vi "map wall setting.vi"(8 "error in (no error)":errorcluster, 11 "wall settings":cluster{"Array":cluster{"X":dbl, "Y":dbl}[]}[](array[cluster])) -> (0 "error out":errorcluster, 3 "<JSON>":string)   [LabVIEW 2019]
uses:
  <vilib>/JDP Science/JSONtext/support/Format JSON Object.vi
  <vilib>/JDP Science/JSONtext/support/Format JSON Array Text.vi
  <vilib>/JDP Science/JSONtext/JSONtext.lvlib
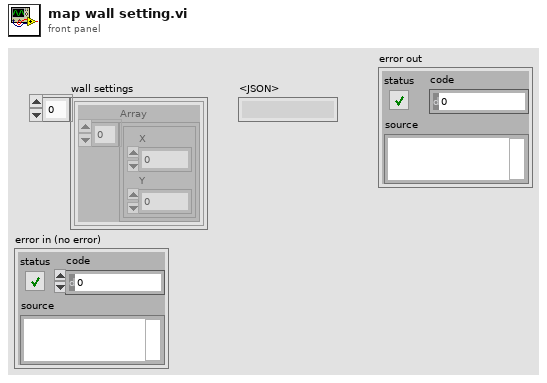
[diagram p1: front panel]
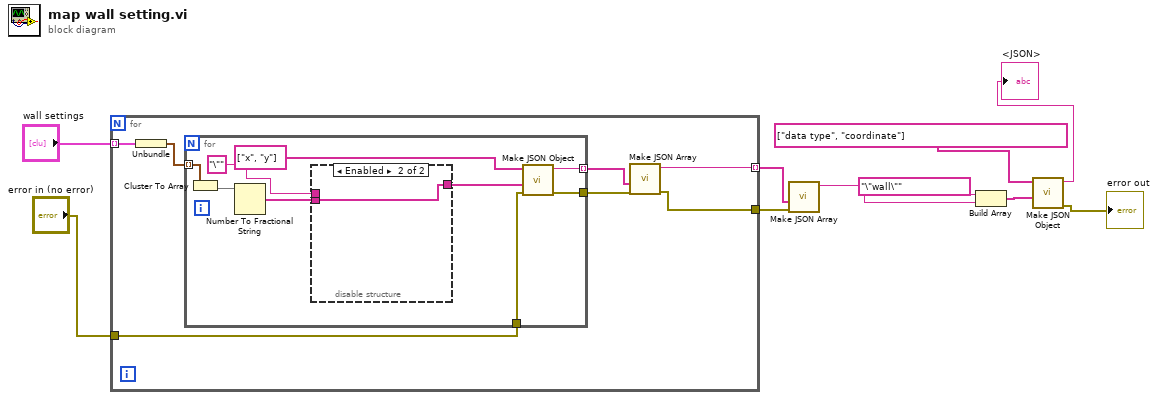
[diagram p0: block diagram]
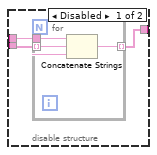
[diagram p2: hidden frame]
diagram:
  n1 = for {
    tunnel: "wall settings" -> [w17] mode=indexing
    tunnel: [w14] -> w10 mode=indexing
    tunnel: "error in (no error)" -> [w13]
    tunnel: [w11] -> w7
    n2 = Unbundle(w17) -> ("Array"=w16:cluster{"X":dbl, "Y":dbl}[])
    n3 = for {
      tunnel: w16 -> [w26] mode=indexing
      tunnel: [w23] -> w15 mode=indexing
      tunnel: w13 -> [w22]
      tunnel: [w21] -> w12
      n4 = Cluster To Array(cluster=w26) -> (array=w25:dbl[])
      n5 = Number To Fractional String(number=w25) -> (F-format string=w20:string[])  [unwired: 3 in]
      n6 = disable-structure shown="Enabled" {
        disable-tunnel: w20 -> [w29 w33]
        disable-tunnel: "\"" -> [w28 _]
        disable-tunnel: [w27 w33] -> w18
        frame Disabled {
          n7 = for {
            tunnel: w29 -> [w32] mode=indexing
            tunnel: w28 -> [w31]
            tunnel: [w30] -> w27 mode=indexing
            n8 = Concatenate Strings(w31, w32, w31) -> (w30:string)
          }
        }
        frame Enabled {
        }
      }
      n9 = call <vilib>:"Make JSON Object.vi"("error in (no error)"=w22, "JSON Items"=w18, "Item Names"=string[] ["x", "y"]) -> ("error out"=w21:errorcluster, "<JSON>"=w23:string)  [unwired: 7 in]
    }
    n10 = call <vilib>:"Make JSON Array.vi"("error in (no error)"=w12, "JSON Elements"=w15) -> ("error out"=w11:errorcluster, "<JSON>"=w14:string)  [unwired: 8 in]
  }
  n11 = call <vilib>:"Make JSON Array.vi"("error in (no error)"=w7, "JSON Elements"=w10) -> ("<JSON>"=w3:string)  [unwired: 8 in, 1 out]
  n12 = Build Array("\"wall\"" ("element"), w3) -> (w4:string[])
  n13 = call <vilib>:"Make JSON Object.vi"("JSON Items"=w4, "Item Names"=string[] ["data type", "coordinate"]) -> ("error out"=→"error out":errorcluster, "<JSON>"=→"<JSON>":string)  [unwired: 8 in]
